vi "LIA7230_Open_Queue.vi"(3 "error in (no error)":errorcluster) -> (0 "error out":errorcluster, 2 "queue out":refnum<queue>)   [LabVIEW 2019]
uses:
  LIA7230/LIA7230-cluster.ctl
  Global/Global Variables/Queues_global.vi
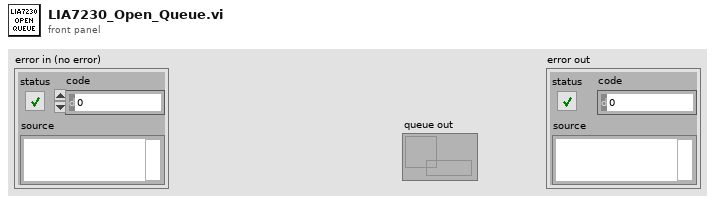
[diagram p1: front panel]
types:
  T1 = typedef "LIA7230-cluster.ctl" = cluster{"Lockin 1":dbl[][], "X1-Display":dbl, "X1 Percent":dbl, "Y1-Display":dbl, "X1 Percent 2":dbl, "Unit X1":string, "Unit X2":string, "X1 Overload":bool, "Y1 Overload":bool, "Sensitivity Setpoint":i16, "X1":dbl, "Y1":dbl, "Channel 3":dbl, "Channel 4":dbl, "Channel 4 Percent":dbl, "Channel 3 Percent ":dbl, "Unit Channel 3":string, "Unit Channel 4":string, "Overload channel 3":bool, "Overload channel 4":bool, "Offsets (ON)":bool, "Sensitivity Setpoint 2":i16}
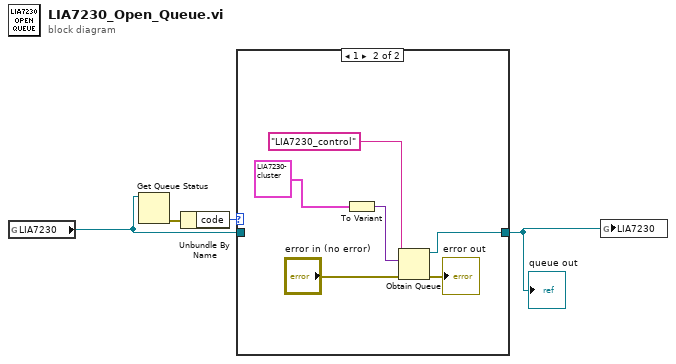
[diagram p0: block diagram]
diagram:
  n1 = global read "Queues_global.vi" "LIA7230"() -> (w2:refnum<queue>)
  n2 = Get Queue Status(queue=w2) -> (error out=w4:errorcluster)  [unwired: 2 in, 7 out]
  n3 = Unbundle By Name(w4) -> ("code"=w3:i32)
  n4 = case shown="1" w3 {
    tunnel: [w5 w7] -> w1
    tunnel: w2 -> [w5 _]
    frame 0, Default {
    }
    frame 1 {
      n5 = To Variant(anything=T1 {"Lockin 1"=[], "X1-Display"=0.0, "X1 Percent"=0.0, "Y1-Display"=0.0, "X1 Percent 2"=0.0, "Unit X1"="nV", "Unit X2"="nV", "X1 Overload"=FALSE, "Y1 Overload"=FALSE, "Sensitivity Setpoint"=26, "X1"=0.0, "Y1"=0.0, "Channel 3"=0.0, "Channel 4"=0.0, "Channel 4 Percent"=0.0, "Channel 3 Percent "=0.0, "Unit Channel 3"="nV", "Unit Channel 4"="nV", "Overload channel 3"=FALSE, "Overload channel 4"=FALSE, "Offsets (ON)"=FALSE, "Sensitivity Setpoint 2"=26} ("LIA7230-Cluser")) -> (Variant=w10:variant)
      n6 = Obtain Queue(name (unnamed)="LIA7230_control", element data type=w10, error in (no error)="error in (no error)") -> (queue out=w7:refnum<queue>, error out=→"error out":errorcluster)  [unwired: 2 in, 1 out]
    }
  }
  "queue out" <- w1
  n7 = global write "Queues_global.vi" "LIA7230"(w1) -> ()
